vi "MenuNameFromTag.vi"(8 "error in (no error)":errorcluster, 10 "item tag":string, 11 "menu reference":refnum<k9>) -> (0 "error out":errorcluster, 2 "item name":string, 3 "menu reference out":refnum<k9>)   [LabVIEW 2013]
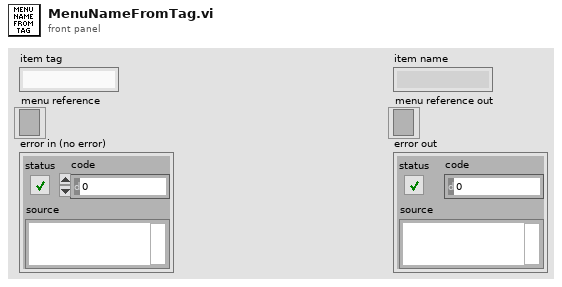
[diagram p1: front panel]
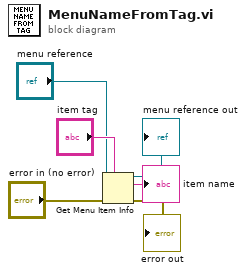
[diagram p0: block diagram]
diagram:
  n1 = Get Menu Item Info(7:"item tag", 8:"error in (no error)", 11:"menu reference") -> (0:→"error out":errorcluster, 2:→"item name":string, 3:→"menu reference out":refnum<k9>)  [unwired: 4 out]
